vi "StopIR.vi"() -> ()   [LabVIEW 2017]
panel:
  out "Stop IR (global)":bool
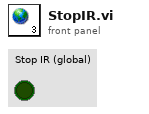
[diagram p1: front panel]
diagram:
